vi "DisposeCore.vi"(8 "error in (no error)":errorcluster, 11 "EnchantedMazeGame":refnum<class "EnchantedMazeGame.lvclass">) -> (0 "error out":errorcluster, 3 "EnchantedMazeGame":refnum<class "EnchantedMazeGame.lvclass">)   [LabVIEW 2020, in "FactoryMethod.lvlib" / "NoParametrizedFactoryMethod.lvlib" / "EnchantedMazeGame.lvclass"]
uses:
  EnchantedMazeGame.lvclass
  Private/TypeDef/privateDataDVR.ctl
  Private/TypeDef/privateData.ctl
  EnchantedMazeGame.lvclass/EnchantedMazeGame.ctl
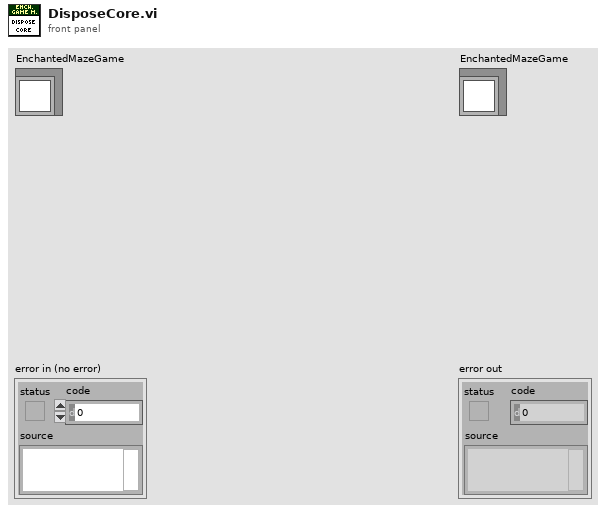
[diagram p1: front panel]
types:
  T1 = typedef "FactoryMethod.lvlib/NoParametrizedFactoryMethod.lvlib/EnchantedMazeGame.lvclass/privateDataDVR.ctl" = refnum<data-value>
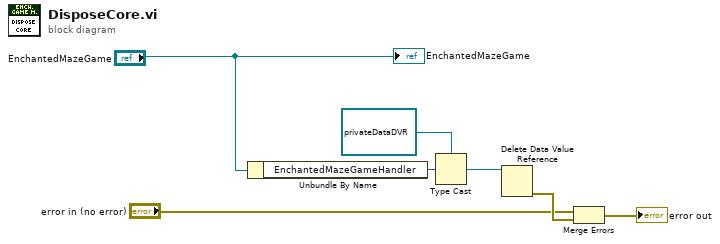
[diagram p0: block diagram]
diagram:
  n1 = Unbundle By Name("EnchantedMazeGame") -> ("EnchantedMazeGameHandler"=w6:u32)
  n2 = Type Cast(type=T1 refnum ("privateDataDVR"), x=w6) -> (*(type *) &x=w7:T1)
  n3 = Delete Data Value Reference(data value reference=w7) -> (error out=w5:errorcluster)  [unwired: 1 in, 1 out]
  n4 = Merge Errors("error in (no error)", w5) -> (→"error out":errorcluster)
  "EnchantedMazeGame" <- "EnchantedMazeGame"
